vi "Upload.vi"   [LabVIEW 2020, in "NI_SFTP.lvlib"]
doc: "Creates multiple remote files. The instance VI determines how the file contents are initialized."
uses:
  <vilib>/net/SFTP/NI_SFTP.lvlib
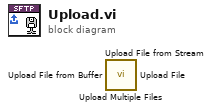
[diagram p0: block diagram]
diagram:
  n1 = call <vilib>:"Upload Multiple Files.vi"() -> ()  [unwired: 10 in, 2 out]
  n2 = call <vilib>:"Upload File from Stream.vi"() -> ()  [unwired: 10 in, 2 out]
  n3 = call <vilib>:"Upload File from Buffer.vi"() -> ()  [unwired: 10 in, 2 out]
  n4 = call <vilib>:"Upload File.vi"() -> ()  [unwired: 10 in, 2 out]
